vi "TCP-IP Link.Rcv Status.vi"(10 "Data":variant) -> (1 "error out":errorcluster, 2 "Status":T1)   [LabVIEW 2024, in "EQMF.lvlib" / "TCP-IP.lvlib"]
uses:
  TCP-IP.lvlib
  Controls/TCP-IP Link.Status.ctl
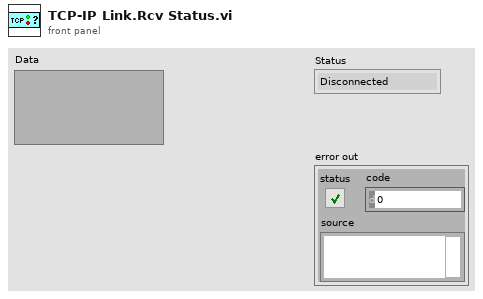
[diagram p1: front panel]
types:
  T1 = typedef "EQMF.lvlib/TCP-IP.lvlib/TCP-IP Link.Status.ctl" = enum16{"Disconnected", "Connected", "Connecting", "Failed to Connect", "Listening"}
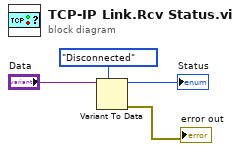
[diagram p0: block diagram]
diagram:
  n1 = Variant To Data(type=TCP-IP_Link.Status."Disconnected" ("Status"), Variant="Data") -> (data=→"Status":T1, error out=→"error out":errorcluster)  [unwired: 1 in]
